vi "Three_Tote_Did_Not_Work_2_15.vi"(11 "3_Tote_Enable":bool) -> ()   [LabVIEW 2014]
uses:
  General_VI/Global Var.vi
panel:
  in  "Reset_Auto":bool
  in  "Time _To_Drive_1_Tote":i32=80000
  in  "Extend_Flipper_Time":i32=500
  in  "Open_Infeed_time":i32=800
  # "Static Tunning Values"
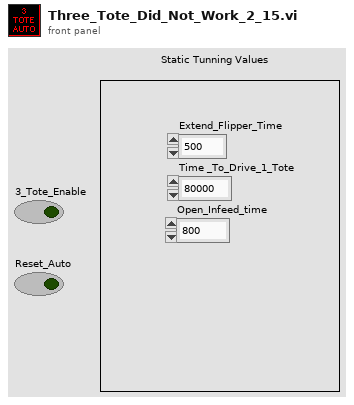
[diagram p1: front panel]
types:
  T1 = cluster{"Open_Infeed_time":i32, "Extend_Flipper_Time":i32, "Time _To_Drive_1_Tote":i32}
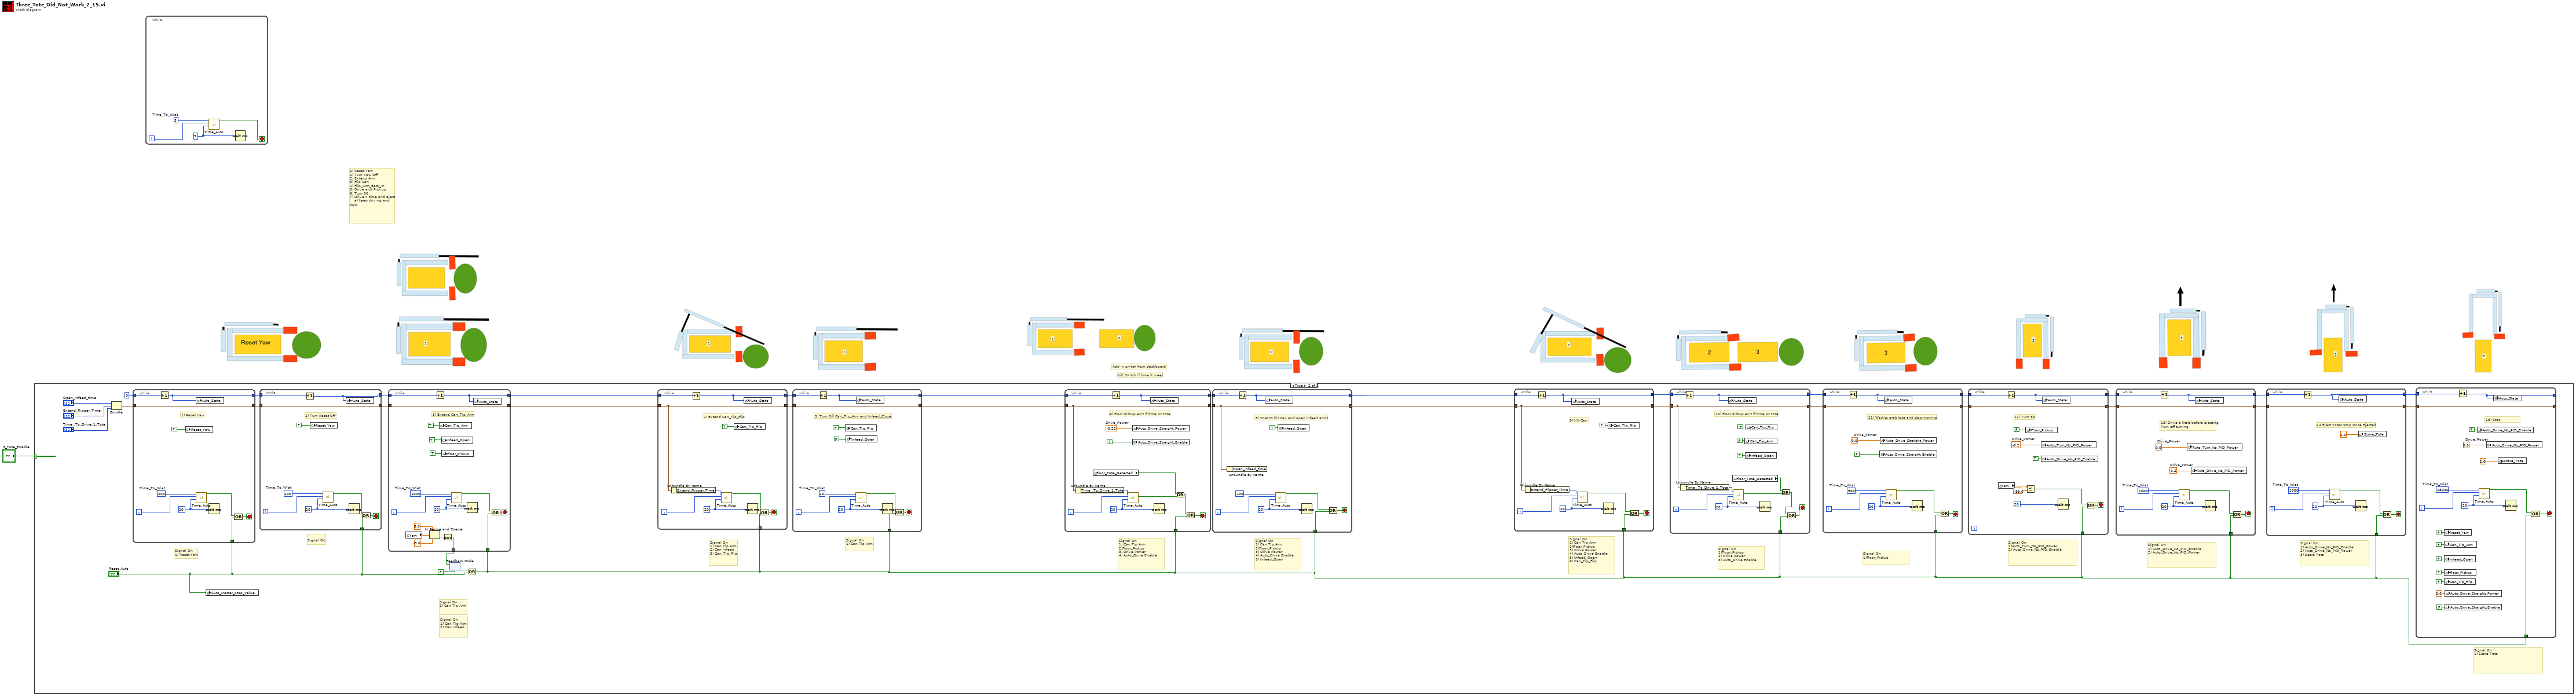
[diagram p0: block diagram]
diagram:
  # "3"
  # "3"
  # "3"
  # "3"
  # "2"
  # "2"
  # "2"
  # "1"
  # "1"
  # "1"
  # "1"
  # "Add in switch from dashboard"
  # "Kill Switch if time it meet"
  # "1) Reset Yaw\n2) Turn Yaw Off\n2) Extend Arm\n3) Flip Can\n4) Flip_Arm_Back_In\n5) Drive and Pick up\n6) Turn 90\n7) Drive x time and eject\n    a) keep driving and      stop"
  n1 = case shown="True" "3_Tote_Enable" {
    frame False {
    }
    frame True {
      # "Signal On\n1) Score Tote"
      # "Signal On\n1) Auto_Drive_No_PID_Enable\n2) Auto_Drive_No_PID_Power\n3) Score Tote"
      # "Signal On\n1) Auto_Drive_No_PID_Enable\n2) Auto_Drive_No_PID_Power"
      # "Signal On\n1)Auto_Turn_No_PID_Power\n2) Auto_Drive_No_PID_Enable"
      # "Signal On\n1)Floor_Pickup"
      # "Signal On\n1)Floor_Pickup\n2) Drive Power\n3) Auto_Drive Enable"
      # "Signal On\n1) Can Tip Arm\n2)Floor_Pickup\n3) Drive Power\n4) Auto_Drive Enable\n5) Infeed_Open\n6) Can_Tip_Flip"
      # "Signal On\n1) Can Tip Arm\n2)Floor_Pickup\n3) Drive Power\n4) Auto_Drive Enable\n5) Infeed_Open"
      # "Signal On\n1) Can Tip Arm\n2)Floor_Pickup\n3) Drive Power\n4) Auto_Drive Enable"
      # "Signal On\n1) Can Tip Arm"
      # "Signal On\n1) Can Tip Arm\n2) Can Infeed\n3) Can_Tip_Flip"
      # "Signal On\n1) Can Tip Arm\n2) Can Infeed"
      # "Signal On\n1) Can Tip Arm"
      # "Signal On"
      # "Signal On\n1) Reset Yaw"
      n2 = Bundle("Open_Infeed_time"="Open_Infeed_time", "Extend_Flipper_Time"="Extend_Flipper_Time", "Time _To_Drive_1_Tote"="Time _To_Drive_1_Tote") -> (w21:T1)  [unwired: 1 in]
      n3 = while {
        tunnel: 0 -> [w200]
        tunnel: [w199] -> w36
        tunnel: w21 -> [w201]
        tunnel: [w201] -> w20
        tunnel: "Reset_Auto" -> [w196]
        i -> [w204]
        stop <- w198 stop-if-true
        w205 = u32 20 ("milliseconds to wait")
        w203 = 200  # Time_To_Wiat
        # "1) Reset Yaw"
        n4 = Increment(x=w200) -> (x+1=w199:i32)
        n5 = global write "Global Var.vi" "Reset_Yaw"(TRUE) -> ()
        n6 = global write "Global Var.vi" "Auto_State"(w199) -> ()
        n7 = call "Time_Auto.vi"("Sample_Time"=w205, "Counter"=w204, "Time_to_wait"=w203) -> ("Boolean"=w197:bool)  [unwired: 8 in]
        n8 = Wait (ms)(milliseconds to wait=w205) -> ()  [unwired: 1 out]
        n9 = Compound Arithmetic op=OR(w197, w196) -> (w198:bool)
      }
      n10 = global write "Global Var.vi" "Auto_Master_Stop_Value"("Reset_Auto") -> ()
      n11 = while {
        tunnel: w36 -> [w190]
        tunnel: [w189] -> w35
        tunnel: w20 -> [w191]
        tunnel: [w191] -> w19
        tunnel: "Reset_Auto" -> [w186]
        i -> [w194]
        stop <- w188 stop-if-true
        w195 = u32 20 ("milliseconds to wait")
        w193 = 200  # Time_To_Wiat
        # "2) Turn Reset Off"
        n12 = Increment(x=w190) -> (x+1=w189:i32)
        n13 = global write "Global Var.vi" "Reset_Yaw"(FALSE) -> ()
        n14 = call "Time_Auto.vi"("Sample_Time"=w195, "Counter"=w194, "Time_to_wait"=w193) -> ("Boolean"=w187:bool)  [unwired: 8 in]
        n15 = global write "Global Var.vi" "Auto_State"(w189) -> ()
        n16 = Wait (ms)(milliseconds to wait=w195) -> ()  [unwired: 1 out]
        n17 = Compound Arithmetic op=OR(w187, w186) -> (w188:bool)
      }
      n18 = feedback #1(FALSE) -> (w3:bool)
      n19 = Or(x=w3, y="Reset_Auto") -> (x .or. y?=w5:bool)
      n20 = while {
        tunnel: w35 -> [w180]
        tunnel: [w179] -> w8
        tunnel: w19 -> [w181]
        tunnel: [w181] -> w7
        tunnel: [w170] -> w4
        tunnel: w5 -> [w169]
        i -> [w184]
        stop <- w176 stop-if-true
        w185 = u32 20 ("milliseconds to wait")
        w183 = 1000  # Time_To_Wiat
        # "3) Extend Can_Tip_Arm"
        n21 = global read "Global Var.vi" "Yaw"() -> (w174:dbl)
        n22 = In Range and Coerce(upper limit=-5.0, x=w174, lower limit=5.0) -> (In Range?=w171:bool)  [unwired: 1 out]
        n23 = Increment(x=w180) -> (x+1=w179:i32)
        n24 = global write "Global Var.vi" "Can_Tip_Arm"(TRUE) -> ()
        n25 = global write "Global Var.vi" "Infeed_Open"(TRUE) -> ()
        n26 = global write "Global Var.vi" "Floor_Pickup"(TRUE) -> ()
        n27 = Not(x=w171) -> (.not. x?=w170:bool)
        n28 = call "Time_Auto.vi"("Sample_Time"=w185, "Counter"=w184, "Time_to_wait"=w183) -> ("Boolean"=w175:bool)  [unwired: 8 in]
        n29 = Wait (ms)(milliseconds to wait=w185) -> ()  [unwired: 1 out]
        n30 = global write "Global Var.vi" "Auto_State"(w179) -> ()
        n31 = Compound Arithmetic op=OR(w175, w169) -> (w176:bool)
      }
      n32 = feedback-in #1(w4) -> ()
      n33 = while {
        tunnel: w8 -> [w165]
        tunnel: [w164] -> w34
        tunnel: w7 -> [w163]
        tunnel: [w163] -> w18
        tunnel: w5 -> [w159]
        i -> [w167]
        stop <- w161 stop-if-true
        w168 = u32 20 ("milliseconds to wait")
        # "4) Extend Can_Tip_Flip"
        n34 = Unbundle By Name(w163) -> ("Extend_Flipper_Time"=w162:i32)
        n35 = Increment(x=w165) -> (x+1=w164:i32)
        n36 = call "Time_Auto.vi"("Sample_Time"=w168, "Counter"=w167, "Time_to_wait"=w162) -> ("Boolean"=w160:bool)  [unwired: 8 in]
        n37 = global write "Global Var.vi" "Can_Tip_Flip"(TRUE) -> ()
        n38 = global write "Global Var.vi" "Auto_State"(w164) -> ()
        n39 = Wait (ms)(milliseconds to wait=w168) -> ()  [unwired: 1 out]
        n40 = Compound Arithmetic op=OR(w160, w159) -> (w161:bool)
      }
      n41 = while {
        tunnel: w34 -> [w152]
        tunnel: [w151] -> w30
        tunnel: w18 -> [w153]
        tunnel: [w153] -> w17
        tunnel: w5 -> [w148]
        i -> [w157]
        stop <- w150 stop-if-true
        w158 = u32 20 ("milliseconds to wait")
        w156 = 20  # Time_To_Wiat
        # "5) Turn Off Can_Flip_Arm and Infeed_Close"
        n42 = Increment(x=w152) -> (x+1=w151:i32)
        n43 = global write "Global Var.vi" "Can_Tip_Flip"(FALSE) -> ()
        n44 = global write "Global Var.vi" "Infeed_Open"(FALSE) -> ()
        n45 = call "Time_Auto.vi"("Sample_Time"=w158, "Counter"=w157, "Time_to_wait"=w156) -> ("Boolean"=w149:bool)  [unwired: 8 in]
        n46 = global write "Global Var.vi" "Auto_State"(w151) -> ()
        n47 = Wait (ms)(milliseconds to wait=w158) -> ()  [unwired: 1 out]
        n48 = Compound Arithmetic op=OR(w149, w148) -> (w150:bool)
      }
      n49 = while {
        tunnel: w30 -> [w143]
        tunnel: [w142] -> w33
        tunnel: w17 -> [w141]
        tunnel: [w141] -> w16
        tunnel: w5 -> [w135]
        i -> [w146]
        stop <- w137 stop-if-true
        w139 = -0.22  # Drive_Power
        w147 = u32 20 ("milliseconds to wait")
        # "6) Floor Pickup exit if time or Tote"
        n50 = Unbundle By Name(w141) -> ("Time _To_Drive_1_Tote"=w140:i32)
        n51 = global read "Global Var.vi" "Floor_Tote_Detected"() -> (w144:bool)
        n52 = Increment(x=w143) -> (x+1=w142:i32)
        n53 = call "Time_Auto.vi"("Sample_Time"=w147, "Counter"=w146, "Time_to_wait"=w140) -> ("Boolean"=w145:bool)  [unwired: 8 in]
        n54 = global write "Global Var.vi" "Auto_Drive_Straight_Enable"(TRUE) -> ()
        n55 = global write "Global Var.vi" "Auto_Drive_Straight_Power"(w139) -> ()
        n56 = global write "Global Var.vi" "Auto_State"(w142) -> ()
        n57 = Wait (ms)(milliseconds to wait=w147) -> ()  [unwired: 1 out]
        n58 = Or(x=w144, y=w145) -> (x .or. y?=w136:bool)
        n59 = Compound Arithmetic op=OR(w136, w135) -> (w137:bool)
      }
      n60 = while {
        tunnel: w33 -> [w131]
        tunnel: [w130] -> w29
        tunnel: w16 -> [w129]
        tunnel: [w129] -> w15
        tunnel: w5 -> [w125]
        i -> [w133]
        stop <- w127 stop-if-true
        w134 = u32 20 ("milliseconds to wait")
        # "8) Wiat to hit Can and open infeed arms"
        n61 = Unbundle By Name(w129) -> ()  [unwired: 1 out]
        n62 = Increment(x=w131) -> (x+1=w130:i32)
        n63 = global write "Global Var.vi" "Auto_State"(w130) -> ()
        n64 = call "Time_Auto.vi"("Sample_Time"=w134, "Counter"=w133, "Time_to_wait"=400) -> ("Boolean"=w126:bool)  [unwired: 8 in]
        n65 = global write "Global Var.vi" "Infeed_Open"(TRUE ("Infeed_Open")) -> ()
        n66 = Wait (ms)(milliseconds to wait=w134) -> ()  [unwired: 1 out]
        n67 = Compound Arithmetic op=OR(w126, w125) -> (w127:bool)
      }
      n68 = while {
        tunnel: w29 -> [w121]
        tunnel: [w120] -> w32
        tunnel: w15 -> [w119]
        tunnel: [w119] -> w14
        tunnel: w5 -> [w115]
        i -> [w123]
        stop <- w117 stop-if-true
        w124 = u32 20 ("milliseconds to wait")
        # "9) HIt Can"
        n69 = Unbundle By Name(w119) -> ("Extend_Flipper_Time"=w118:i32)
        n70 = Increment(x=w121) -> (x+1=w120:i32)
        n71 = global write "Global Var.vi" "Auto_State"(w120) -> ()
        n72 = call "Time_Auto.vi"("Sample_Time"=w124, "Counter"=w123, "Time_to_wait"=w118) -> ("Boolean"=w116:bool)  [unwired: 8 in]
        n73 = Wait (ms)(milliseconds to wait=w124) -> ()  [unwired: 1 out]
        n74 = global write "Global Var.vi" "Can_Tip_Flip"(TRUE ("Infeed_Open")) -> ()
        n75 = Compound Arithmetic op=OR(w116, w115) -> (w117:bool)
      }
      n76 = while {
        tunnel: w32 -> [w107]
        tunnel: [w106] -> w31
        tunnel: w14 -> [w104]
        tunnel: [w104] -> w13
        tunnel: w5 -> [w101]
        i -> [w113]
        stop <- w103 stop-if-true
        w114 = u32 20 ("milliseconds to wait")
        # "10) Floor Pickup exit if time or Tote"
        n77 = Unbundle By Name(w104) -> ("Time _To_Drive_1_Tote"=w105:i32)
        n78 = Increment(x=w107) -> (x+1=w106:i32)
        n79 = global write "Global Var.vi" "Auto_State"(w106) -> ()
        n80 = global read "Global Var.vi" "Floor_Tote_Detected"() -> (w111:bool)
        n81 = call "Time_Auto.vi"("Sample_Time"=w114, "Counter"=w113, "Time_to_wait"=w105) -> ("Boolean"=w112:bool)  [unwired: 8 in]
        n82 = global write "Global Var.vi" "Can_Tip_Arm"(FALSE ("Infeed_Open")) -> ()
        n83 = global write "Global Var.vi" "Infeed_Open"(FALSE ("Infeed_Open")) -> ()
        n84 = global write "Global Var.vi" "Can_Tip_Flip"(FALSE ("Infeed_Open")) -> ()
        n85 = Wait (ms)(milliseconds to wait=w114) -> ()  [unwired: 1 out]
        n86 = Or(x=w111, y=w112) -> (x .or. y?=w102:bool)
        n87 = Compound Arithmetic op=OR(w102, w101) -> (w103:bool)
      }
      n88 = while {
        tunnel: w31 -> [w96]
        tunnel: [w95] -> w28
        tunnel: w13 -> [w97]
        tunnel: [w97] -> w12
        tunnel: w5 -> [w90]
        i -> [w99]
        stop <- w92 stop-if-true
        w94 = 0.0  # Drive_Power
        w100 = u32 20 ("milliseconds to wait")
        w98 = 500  # Time_To_Wiat
        # "11) Wait to grab tote and stop moving"
        n89 = Increment(x=w96) -> (x+1=w95:i32)
        n90 = global write "Global Var.vi" "Auto_Drive_Straight_Enable"(FALSE) -> ()
        n91 = global write "Global Var.vi" "Auto_Drive_Straight_Power"(w94) -> ()
        n92 = global write "Global Var.vi" "Auto_State"(w95) -> ()
        n93 = call "Time_Auto.vi"("Sample_Time"=w100, "Counter"=w99, "Time_to_wait"=w98) -> ("Boolean"=w91:bool)  [unwired: 8 in]
        n94 = Wait (ms)(milliseconds to wait=w100) -> ()  [unwired: 1 out]
        n95 = Compound Arithmetic op=OR(w91, w90) -> (w92:bool)
      }
      n96 = while {
        tunnel: w28 -> [w84]
        tunnel: [w83] -> w27
        tunnel: w12 -> [w85]
        tunnel: [w85] -> w11
        tunnel: w5 -> [w78]
        stop <- w79 stop-if-true
        w82 = -0.2  # Drive_Power
        # "12) Turn 90"
        n97 = global read "Global Var.vi" "Yaw"() -> (w87:dbl)
        n98 = Increment(x=w84) -> (x+1=w83:i32)
        n99 = Less Or Equal?(x=w87, y=-85.0) -> (x <= y?=w80:bool)
        n100 = global write "Global Var.vi" "Floor_Pickup"(FALSE) -> ()
        n101 = global write "Global Var.vi" "Auto_Turn_No_PID_Power"(w82) -> ()
        n102 = global write "Global Var.vi" "Auto_Drive_No_PID_Enable"(TRUE ("Auto_Drive_No_PID_Enable")) -> ()
        n103 = global write "Global Var.vi" "Auto_State"(w83) -> ()
        n104 = Wait (ms)(milliseconds to wait=u32 20) -> ()  [unwired: 1 out]
        n105 = Compound Arithmetic op=OR(w80, w78) -> (w79:bool)
      }
      n106 = while {
        tunnel: w27 -> [w72]
        tunnel: [w71] -> w26
        tunnel: w11 -> [w73]
        tunnel: [w73] -> w10
        tunnel: w5 -> [w67]
        i -> [w76]
        stop <- w69 stop-if-true
        w70 = 0.0  # Drive_Power
        w74 = 0.2  # Drive_Power
        w77 = u32 20 ("milliseconds to wait")
        w75 = 1000  # Time_To_Wiat
        # "13) Drive a little before ejecting\nTurn off turning"
        n107 = Increment(x=w72) -> (x+1=w71:i32)
        n108 = call "Time_Auto.vi"("Sample_Time"=w77, "Counter"=w76, "Time_to_wait"=w75) -> ("Boolean"=w68:bool)  [unwired: 8 in]
        n109 = global write "Global Var.vi" "Auto_Turn_No_PID_Power"(w70) -> ()
        n110 = global write "Global Var.vi" "Auto_Drive_No_PID_Power"(w74) -> ()
        n111 = global write "Global Var.vi" "Auto_State"(w71) -> ()
        n112 = Wait (ms)(milliseconds to wait=w77) -> ()  [unwired: 1 out]
        n113 = Compound Arithmetic op=OR(w68, w67) -> (w69:bool)
      }
      n114 = while {
        tunnel: w26 -> [w61]
        tunnel: [w60] -> w25
        tunnel: w10 -> [w62]
        tunnel: [w62] -> w9
        tunnel: w5 -> [w57]
        i -> [w65]
        stop <- w59 stop-if-true
        w66 = u32 20 ("milliseconds to wait")
        w64 = 1000  # Time_To_Wiat
        # "14)Eject Totes Stop Once Ejected"
        n115 = Increment(x=w61) -> (x+1=w60:i32)
        n116 = call "Time_Auto.vi"("Sample_Time"=w66, "Counter"=w65, "Time_to_wait"=w64) -> ("Boolean"=w58:bool)  [unwired: 8 in]
        n117 = global write "Global Var.vi" "Auto_State"(w60) -> ()
        n118 = Wait (ms)(milliseconds to wait=w66) -> ()  [unwired: 1 out]
        n119 = global write "Global Var.vi" "Score_Tote"(1.0) -> ()
        n120 = Compound Arithmetic op=OR(w58, w57) -> (w59:bool)
      }
      n121 = while {
        tunnel: w25 -> [w51]
        tunnel: w9 -> [w52]
        tunnel: [w52] -> _
        tunnel: [w50] -> _
        tunnel: w5 -> [w38]
        i -> [w55]
        stop <- w46 stop-if-true
        w48 = 0.0  # Drive_Power
        w56 = u32 20 ("milliseconds to wait")
        w54 = 15000  # Time_To_Wiat
        # "15) Stop"
        n122 = global write "Global Var.vi" "Reset_Yaw"(FALSE ("Reset_Yaw")) -> ()
        n123 = global write "Global Var.vi" "Can_Tip_Arm"(FALSE ("Can_Tip_Arm")) -> ()
        n124 = global write "Global Var.vi" "Infeed_Open"(FALSE ("Infeed_Open")) -> ()
        n125 = global write "Global Var.vi" "Floor_Pickup"(FALSE ("Floor_Pickup")) -> ()
        n126 = global write "Global Var.vi" "Can_Tip_Flip"(FALSE ("Can_Tip_Flip")) -> ()
        n127 = global write "Global Var.vi" "Auto_Drive_Straight_Enable"(FALSE ("Auto_Drive_Straight_Enable")) -> ()
        n128 = global write "Global Var.vi" "Auto_Drive_Straight_Power"(0.0 ("Auto_Drive_Straight_Power")) -> ()
        n129 = Increment(x=w51) -> (x+1=w50:i32)
        n130 = global write "Global Var.vi" "Auto_Drive_No_PID_Enable"(FALSE ("Auto_Drive_No_PID_Enable")) -> ()
        n131 = call "Time_Auto.vi"("Sample_Time"=w56, "Counter"=w55, "Time_to_wait"=w54) -> ("Boolean"=w47:bool)  [unwired: 8 in]
        n132 = global write "Global Var.vi" "Auto_Drive_No_PID_Power"(w48) -> ()
        n133 = global write "Global Var.vi" "Auto_State"(w50) -> ()
        n134 = global write "Global Var.vi" "Score_Tote"(1.0) -> ()
        n135 = Wait (ms)(milliseconds to wait=w56) -> ()  [unwired: 1 out]
        n136 = Compound Arithmetic op=OR(w47, w38) -> (w46:bool)
      }
    }
  }
  n137 = while {
    i -> [w207]
    stop <- w209 stop-if-true
    w208 = u32 5 ("milliseconds to wait")
    w206 = 5  # Time_To_Wiat
    n138 = call "Time_Auto.vi"("Sample_Time"=w208, "Counter"=w207, "Time_to_wait"=w206) -> ("Boolean"=w209:bool)  [unwired: 8 in]
    n139 = Wait (ms)(milliseconds to wait=w208) -> ()  [unwired: 1 out]
  }
